vi "Get 1D String.vi"(7 "key description":string, 8 "sections":string[](array[string]), 9 "string":string[](array[string]), 11 "info data":string) -> (0 "sections out":string[](array[string]), 1 "key found?":bool, 2 "value":string[](array[string]), 3 "info data out":string)   [LabVIEW 2020, in "infolib.lvlib"]
doc: "Reads horizontal or vertical vector of strings. If section is entered it searches the key in the section(s)."
uses:
  infolib.lvlib
  Get 2D String.vi
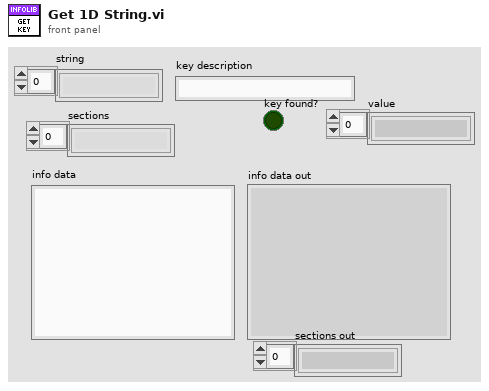
[diagram p1: front panel]
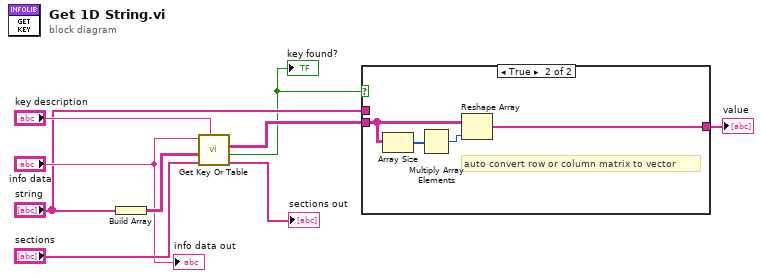
[diagram p0: block diagram]
diagram:
  n1 = Build Array("string") -> (w8:string[][])
  n2 = call-poly "Get Key Or Table.vi"("key description"="key description", "sections"="sections", "string"=w8, "info data"="info data") -> ("sections out"=→"sections out":string[], "key found?"=w1:bool, "value"=w4:string[][])  [unwired: 4 in, 1 out]
  "key found?" <- w1
  n3 = case shown="True" w1 {
    tunnel: [w10 w12] -> w9
    tunnel: w4 -> [_ w11]
    tunnel: "string" -> [w10 _]
    frame False {
    }
    frame True {
      # "auto convert row or column matrix to vector"
      n4 = Array Size(array=w11) -> (size(s)=w14:i32[])
      n5 = Multiply Array Elements(1:w14) -> (0:w13:i32)
      n6 = Reshape Array(w11, w13) -> (w12:string[])
    }
  }
  "value" <- w9
  "info data out" <- "info data"
